vi "WebTestStart.vi"(8 "错误输入（无错误）":errorcluster, 10 "ProductID":string, 11 "client handle":T1 caption="客户端句柄") -> (0 "error Out":errorcluster caption="error IO", 1 "success":bool, 2 "Message":string, 3 "client handle out":T1 caption="客户端句柄输出", 4 "out":string, 5 "input":string)   [LabVIEW 2017]
uses:
  <vilib>/httpClient/LabVIEWHTTPClient.lvlib
  <vilib>/httpClient/POSTBuffer.vi
  <vilib>/httpClient/ClientHandle.ctl
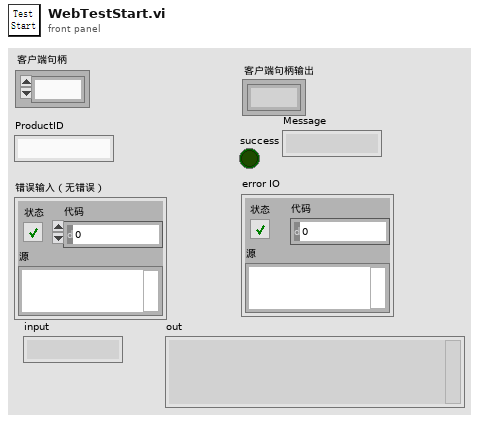
[diagram p1: front panel]
types:
  T1 = typedef "LabVIEWHTTPClient.lvlib/ClientHandle.ctl" = refnum<k1>
  T2 = typedef "HD Config.ctl" = cluster{"ConnectPLC":cluster{"PLC Address":u8[], "PLC Port":i32, "PC Address":u8[]}, "FCO Model 4":cluster{"Com":refnum<visa-resource-name>, "Port":u32}, "FCO Model 7":cluster{"Com":refnum<visa-resource-name>, "Port":u32}, "Flow meter":cluster{"Com":refnum<visa-resource-name>, "Port":u32, "Units":enum16{"Standard", "Volumetric"}}}
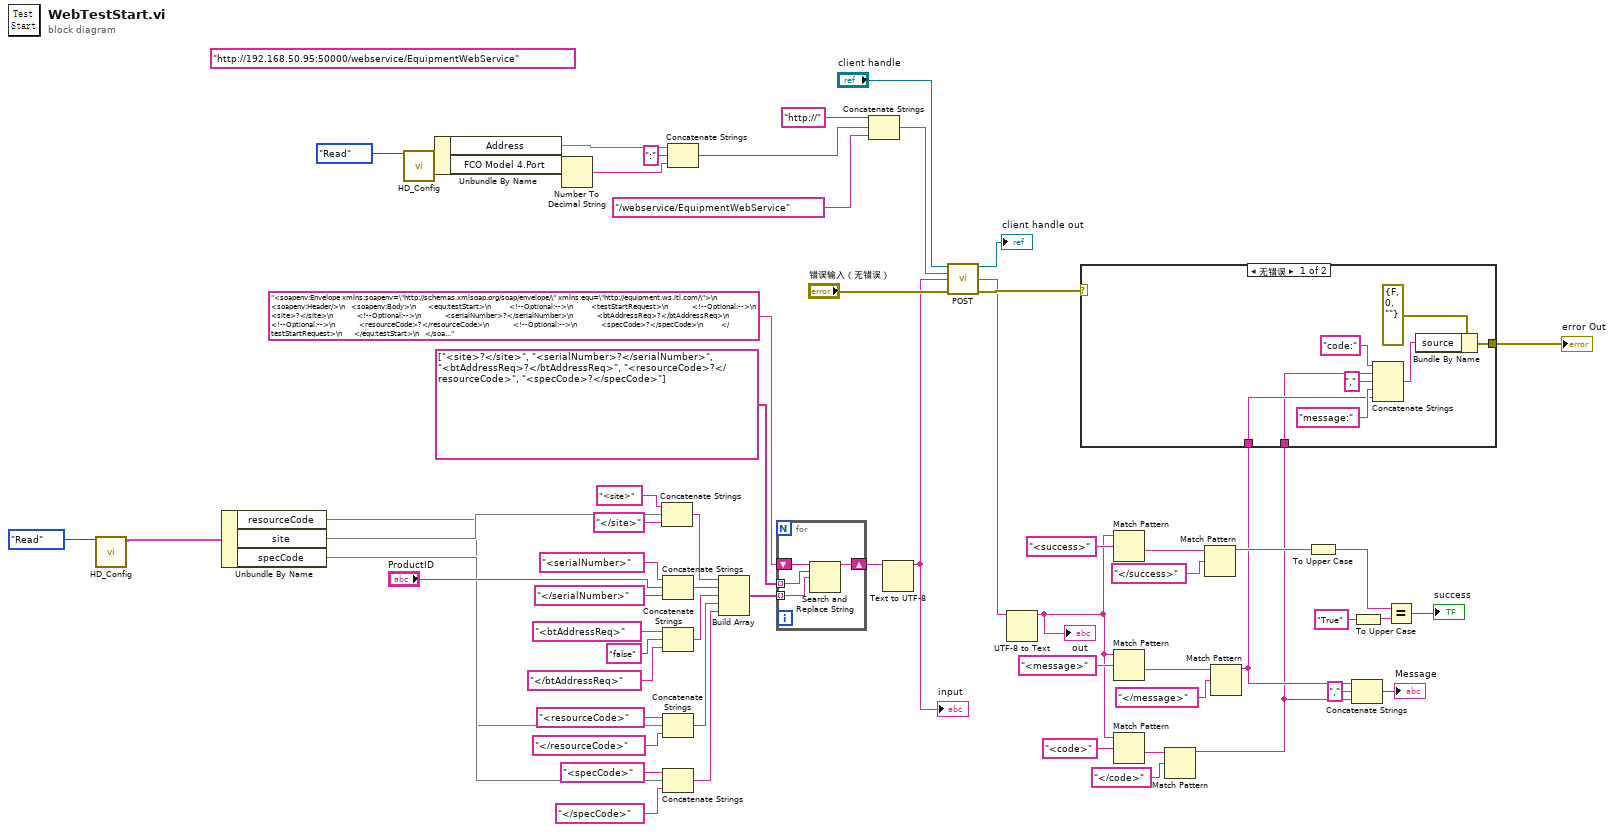
[diagram p0: block diagram]
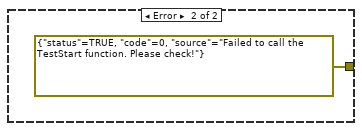
[diagram p2: hidden frame]
diagram:
  (unwired) "http://192.168.50.95:50000/webservice/EquipmentWebService" ("url")
  n1 = call "HD_Config.vi"("Step"=enum16{"Initial", "Write", "Read"}."Read") -> ("HD Config out"=w15:T2)  [unwired: 9 in, 1 out]
  n2 = Unbundle By Name(w15) -> ("resourceCode"=w32, "site"=w35, "specCode"=w33)
  n3 = call "HD_Config.vi"("Step"=enum16{"Initial", "Write", "Read"}."Read") -> ("HD Config out"=w8:T2)  [unwired: 9 in, 1 out]
  n4 = Unbundle By Name(w8) -> ("Address"=w6, "FCO Model 4.Port"=w7:u32)
  n5 = Number To Decimal String(number=w7) -> (decimal integer string=w5:string)  [unwired: 1 in]
  n6 = Concatenate Strings("<site>", w35, "</site>") -> (w44:string)
  n7 = Concatenate Strings("<serialNumber>", "ProductID", "</serialNumber>") -> (w43:string)
  n8 = Concatenate Strings("<btAddressReq>", "false" ("字符串"), "</btAddressReq>") -> (w42:string)
  n9 = Concatenate Strings("<resourceCode>", w32, "</resourceCode>") -> (w41:string)
  n10 = Concatenate Strings("<specCode>", w33, "</specCode>") -> (w40:string)
  n11 = Concatenate Strings(w6, ":" ("字符串"), w5) -> (w2:string)
  n12 = Build Array(w44, w43, w42, w41, w40) -> (w39:string[])
  n13 = for {
    tunnel: string[] ["<site>?</site>", "<serialNumber>?</serialNumber>", "<btAddressReq>?</btAddressReq>", "<resourceCode>?</resourceCode>", "<specCode>?</specCode>"] -> [w64] mode=indexing
    shift-right: [w65] -> w38
    shift-left: "<soapenv:Envelope xmlns:soapenv=\"http://schemas.xmlsoap.org/soap/envelope/\" xmlns:equ=\"http://equipment.ws.itl.com/\">\n   <soapenv:Header/>\n   <soapenv:Body>\n      <equ:testStart>\n         <!--Optional:-->\n         <testStartRequest>\n            <!--Optional:-->\n            <site>?</site>\n            <!--Optional:-->\n            <serialNumber>?</serialNumber>\n            <btAddressReq>?</btAddressReq>\n            <!--Optional:-->\n            <resourceCode>?</resourceCode>\n            <!--Optional:-->\n            <specCode>?</specCode>\n         </testStartRequest>\n      </equ:testStart>\n   </soapenv:Body>\n</soapenv:Envelope>" -> [w66]
    tunnel: w39 -> [w63] mode=indexing
    n14 = Search and Replace String(input string=w66, search string=w64, replace string=w63) -> (result string=w65:string)  [unwired: 5 in, 3 out]
  }
  n15 = Concatenate Strings("http://" ("url"), w2, "/webservice/EquipmentWebService" ("url")) -> (w3:string)
  n16 = Text to UTF-8(11:w38) -> (3:w36:string)  [unwired: 2 in, 1 out]
  "input" <- w36
  n17 = call-poly <vilib>:"POST.vi"("client handle"="client handle", "url"=w3, "buffer"=w36, "error in (no error)"="错误输入（无错误）") -> ("client handle out"=→"client handle out":T1, "body"=w22:string, "error out"=w58:errorcluster)  [unwired: 8 in, 1 out]
  n18 = UTF-8 to Text(11:w22) -> (3:w14:string)  [unwired: 2 in, 1 out]
  "out" <- w14
  n19 = Match Pattern(string=w14, regular expression="<success>") -> (after substring=w24:string)  [unwired: 1 in, 3 out]
  n20 = Match Pattern(string=w14, regular expression="<message>") -> (after substring=w27:string)  [unwired: 1 in, 3 out]
  n21 = Match Pattern(string=w14, regular expression="<code>") -> (after substring=w30:string)  [unwired: 1 in, 3 out]
  n22 = Match Pattern(string=w30, regular expression="</code>") -> (before substring=w12:string)  [unwired: 1 in, 3 out]
  n23 = Match Pattern(string=w24, regular expression="</success>") -> (before substring=w20:string)  [unwired: 1 in, 3 out]
  n24 = Match Pattern(string=w27, regular expression="</message>") -> (before substring=w13:string)  [unwired: 1 in, 3 out]
  n25 = case shown="无错误" w58 {
    tunnel: [w69 errorcluster {"status"=TRUE, "code"=0, "source"="Failed to call the TestStart function. Please check!"} ("error IO")] -> w62
    tunnel: w13 -> [w68 _]
    tunnel: w12 -> [w67 _]
    frame No Error {
      n26 = Concatenate Strings("code:" ("字符串"), w67, "," ("字符串"), "message:" ("字符串"), w68) -> (w71:string)
      n27 = Bundle By Name(cluster=errorcluster {"status"=FALSE, "code"=0, "source"=""} ("error IO"), "source"=w71) -> (w69:errorcluster)
    }
    frame Error {
    }
  }
  "error Out" <- w62
  n28 = To Upper Case(1:w20) -> (0:w19:string)
  n29 = Concatenate Strings(w13, "," ("string"), w12) -> (→"Message":string)
  n30 = To Upper Case(1:"True" ("子字符串之前")) -> (0:w18:string)
  n31 = Equal?(x=w19, y=w18) -> (x = y?=→"success":bool)
